vi "removeComponent.vi"(0 "HGF_Composite":refnum<class "HGF_Composite.lvclass">, 2 "objectName":string, 3 "objectIndex":i32, 5 "error in (no error)":errorcluster) -> (14 "dup HGF_Composite":refnum<class "HGF_Composite.lvclass">, 16 "HGF_Component":refnum<class "HGF_Component.lvclass">, 19 "error out":errorcluster)   [LabVIEW 2014, in "HGF_BaseClasses.lvlib" / "HGF_Composite.lvclass"]
doc: "Remove a Component object from Composite object.\n\nYou can specify either objectName or objectIndex.\nIf objectName is empty string the objectIndex will be used."
uses:
  HGF_Composite.lvclass
  HGF_Component/HGF_Component.lvclass
  HGF_Factory/HGF_Factory.lvclass
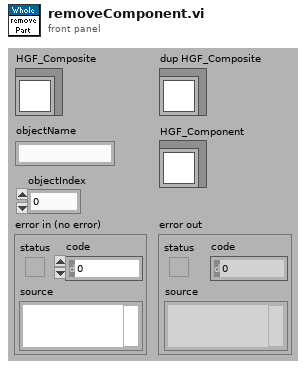
[diagram p1: front panel]
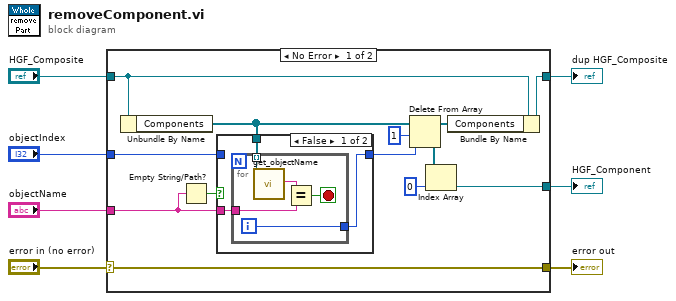
[diagram p0: block diagram]
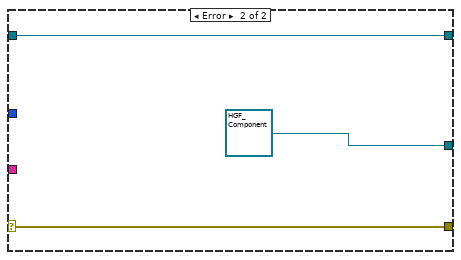
[diagram p3: hidden frame]
diagram:
  n1 = case shown="No Error" "error in (no error)" {
    selector: "error in (no error)" -> [w20 w32]
    tunnel: [w20 w32] -> w6
    tunnel: [w18 w31] -> w4
    tunnel: "HGF_Composite" -> [w19 w31]
    tunnel: "objectIndex" -> [w10 _]
    tunnel: [w13 refnum<class "HGF_Component.lvclass"> refnum ("HGF_Component.lvclass")] -> w2
    tunnel: "objectName" -> [w8 _]
    frame No Error {
      n2 = Unbundle By Name(w19) -> ("Components"=w12:refnum<class "HGF_Component.lvclass">[])
      n3 = Empty String/Path?(string/path=w8) -> (empty?=w9:bool)
      n4 = case shown="False" w9 {
        tunnel: w12 -> [w23 _]
        tunnel: w8 -> [w22 _]
        tunnel: [w21 w29] -> w11
        tunnel: w10 -> [_ w29]
        frame False {
          n5 = for {
            tunnel: w23 -> [w28] mode=indexing
            tunnel: w22 -> [w25]
            tunnel: [w24] -> w21
            i -> [w24]
            stop <- w27 stop-if-true
            n6 = call "get_objectName.vi"("HGF_Factory"=w28) -> ("objectName"=w26:string)  [unwired: 1 in, 17 out]
            n7 = Equal?(x=w26, y=w25) -> (x = y?=w27:bool)
          }
        }
        frame True {
        }
      }
      n8 = Delete From Array(array=w12, length=1, index=w11) -> (deleted portion=w16:refnum<class "HGF_Component.lvclass">[], array with subset deleted=w17:refnum<class "HGF_Component.lvclass">[])
      n9 = Index Array(array=w16, index=0) -> (element=w13:refnum<class "HGF_Component.lvclass">)
      n10 = Bundle By Name(cluster=w19, "Components"=w17) -> (w18:refnum<class "HGF_Composite.lvclass">)
    }
    frame Error {
    }
  }
  "error out" <- w6
  "dup HGF_Composite" <- w4
  "HGF_Component" <- w2
